vi "Uniform Random.vi"(6 "seed":i32=-1, 7 "reset":bool, 9 "xmax":dbl=1.0, 10 "xmin":dbl, 11 "samples":i32=128) -> (0 "error":i32, 3 "uniform random data":dbl[](array[numeric]))   [LabVIEW 2017, in "NI_Gmath.lvlib"]
doc: "Generates random values from a variate X, where X describes the selected distribution type. You must manually select the polymorphic instance to use."
uses:
  NI_Gmath.lvlib
  st_error_code.ctl
  NI_AALBase.lvlib
panel:
  # "Uniform Random"
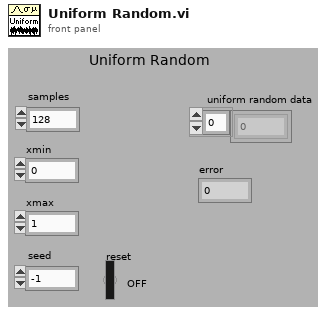
[diagram p1: front panel]
types:
  T1 = typedef "NI_Gmath.lvlib/st_error_code.ctl" = i32
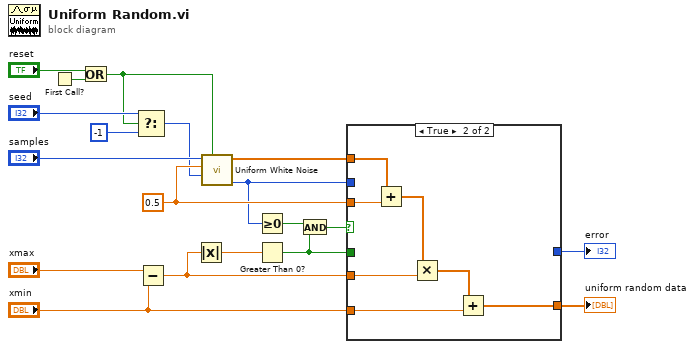
[diagram p0: block diagram]
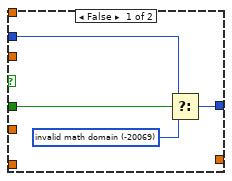
[diagram p2: hidden frame]
diagram:
  w17 = 0.5 ("amplitude")
  n1 = First Call?() -> (First Call?: T/F=w14:bool)
  n2 = Or(x="reset", y=w14) -> (x .or. y?=w9:bool)
  n3 = Select(t="seed", s=w9, f=-1) -> (s? t:f=w10:i32)
  n4 = Subtract(x="xmax", y="xmin") -> (x-y=w4:dbl)
  n5 = Absolute Value(x=w4) -> (abs(x)=w7:dbl)
  n6 = call "Uniform White Noise.vi"("initialize?"=w9, "seed"=w10, "amplitude"=w17, "samples"="samples") -> ("error"=w8:i32, "uniform white noise"=w18:dbl[])  [unwired: 6 in]
  n7 = Greater Or Equal To 0?(x=w8) -> (x >= 0?=w2:bool)
  n8 = Greater Than 0?(x=w7) -> (x > 0?=w1:bool)
  n9 = And(x=w2, y=w1) -> (x .and. y?=w3:bool)
  n10 = case shown="True" w3 {
    tunnel: w18 -> [_ w30]
    tunnel: w17 -> [_ w29]
    tunnel: "xmin" -> [_ w26]
    tunnel: w4 -> [_ w25]
    tunnel: [_ w24] -> w16
    tunnel: [w22 _] -> w15
    tunnel: w8 -> [w21 _]
    tunnel: w1 -> [w23 _]
    frame False {
      w20 = T1 -20069 items=["invalid math domain"=-20069, "Fourier interpolation size m >= n"=-20070, "empty array"=-20003] ("stat interp error code")
      n11 = Select(t=w21, s=w23, f=w20) -> (s? t:f=w22:T1)
    }
    frame True {
      n12 = Add(x=w30, y=w29) -> (x+y=w27:dbl[])
      n13 = Multiply(x=w27, y=w25) -> (x*y=w28:dbl[])
      n14 = Add(x=w28, y=w26) -> (x+y=w24:dbl[])
    }
  }
  "error" <- w15
  "uniform random data" <- w16
